vi "Produce_averaged_Rows.vi"(6 "Absisca":u16, 8 "Row numbers":dbl[](array[numeric]), 9 "Tolerances":dbl[](array[numeric]), 10 "Array in":dbl[](array[numeric]), 11 "Data":string[][](array[string])) -> (3 "Array out":string[][](array[string]))   [LabVIEW 2016]
uses:
  Results_plotter_Global.vi
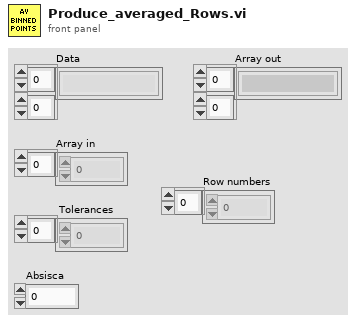
[diagram p1: front panel]
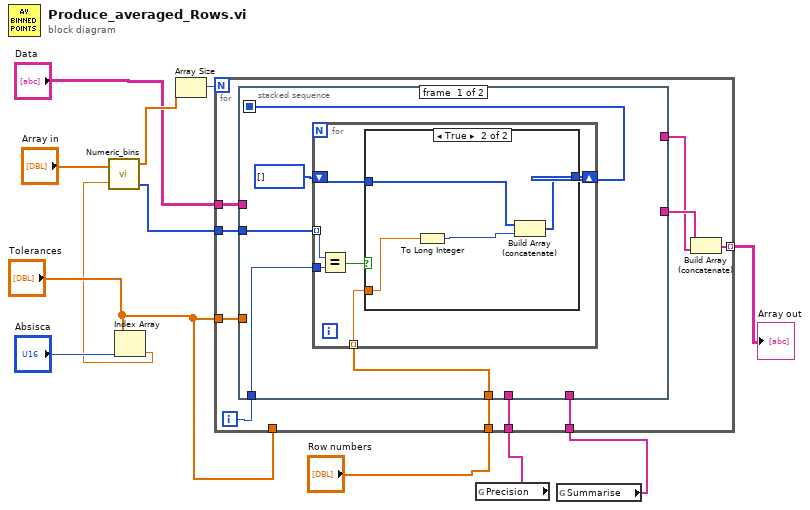
[diagram p0: block diagram]
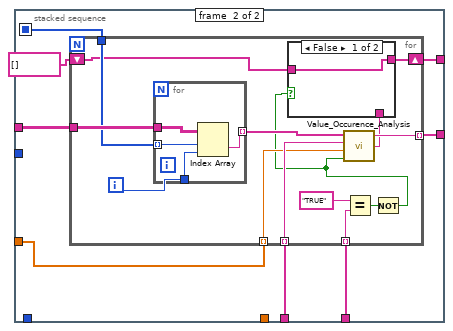
[diagram p3: hidden frame]
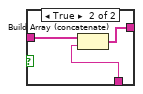
[diagram p4: hidden frame]
diagram:
  n1 = Index Array(array="Tolerances", index="Absisca") -> (element=w7:dbl)
  n2 = call "Numeric_bins.vi"("Values"="Array in", "Tolerance"=w7) -> ("Bin Centres"=w8:dbl[], "Bin Index"=w9:i32[])  [unwired: 1 out]
  n3 = Array Size(array=w8) -> (size(s)=w4:i32)
  n4 = global read "Results_plotter_Global.vi" "Precision"() -> (w5:string[])
  n5 = global read "Results_plotter_Global.vi" "Summarise"() -> (w10:string[])
  n6 = for {
    N: w4 -> [_]
    tunnel: "Data" -> [w22]
    tunnel: w5 -> [w21]
    tunnel: "Tolerances" -> [_]
    tunnel: [w14] -> w3 mode=indexing
    tunnel: w10 -> [w20]
    tunnel: w9 -> [w18]
    tunnel: "Row numbers" -> [w17]
    tunnel: "Tolerances" -> [w13]
    i -> [w19]
    n7 = stacked-sequence {
      seq-local: [w26 _] -> [_ w45]
      tunnel: w22 -> [_ w46]
      tunnel: w21 -> [_ w44]
      tunnel: w20 -> [_ w43]
      tunnel: w19 -> [w25 _]
      tunnel: w18 -> [w24 _]
      tunnel: w17 -> [w23 _]
      tunnel: [_ w41] -> w16
      tunnel: [_ w40] -> w15
      tunnel: w13 -> [_ w39]
      frame #0 {
        n8 = for {
          shift-right: [w32] -> w26
          shift-left: i32[] [] -> [w33]
          tunnel: w25 -> [w31]
          tunnel: w24 -> [w30] mode=indexing
          tunnel: w23 -> [w28] mode=indexing
          n9 = Equal?(x=w30, y=w31) -> (x = y?=w29:bool)
          n10 = case shown="True" w29 {
            tunnel: w33 -> [w34 w37]
            tunnel: [w34 w38] -> w32
            tunnel: w28 -> [_ w35]
            frame False {
            }
            frame True {
              n11 = To Long Integer(number=w35) -> (32bit integer=w36:i32)
              n12 = Build Array (concatenate)(w37, w36) -> (w38:i32[])
            }
          }
        }
      }
      frame #1 {
        n13 = for {
          tunnel: w46 -> [w60]
          tunnel: w45 -> [w59]
          tunnel: w44 -> [w57] mode=indexing
          tunnel: w39 -> [w56] mode=indexing
          tunnel: [w55] -> w41 mode=indexing
          tunnel: w43 -> [w52] mode=indexing
          shift-right: [w47] -> w40
          shift-left: string[] [] -> [w48]
          i -> [w54]
          n14 = for {
            tunnel: w60 -> [w68]
            tunnel: w59 -> [w67] mode=indexing
            tunnel: [w66] -> w58 mode=indexing
            tunnel: w54 -> [w65]
            n15 = Index Array(array=w68, index (row)=w67, index (col)=w65) -> (element=w66:string)
          }
          n16 = Equal?(x="TRUE", y=w52) -> (x = y?=w51:bool)
          n17 = Not(x=w51) -> (.not. x?=w50:bool)
          n18 = call "Value_Occurence_Analysis.vi"("Average Numeric Values?"=w50, "Tolerance"=w56, "Precision (3)"=w57, "String Array"=w58) -> ("St Dev"=w49:string, "Output String"=w55:string)  [unwired: 1 out]
          n19 = case shown="False" w50 {
            tunnel: w49 -> [_ w64]
            tunnel: w48 -> [w61 w63]
            tunnel: [w61 w62] -> w47
            frame False {
            }
            frame True {
              n20 = Build Array (concatenate)(w63, w64) -> (w62:string[])
            }
          }
        }
      }
    }
    n21 = Build Array (concatenate)(w16, w15) -> (w14:string[])
  }
  "Array out" <- w3
